vi "Set Setpoint.vi"(8 "error in":errorcluster, 10 "Setpoint":sgl, 11 "Alicat Controller in":refnum<class "Alicat Controller.lvclass">) -> (0 "error out":errorcluster, 3 "Alicat Controller out":refnum<class "Alicat Controller.lvclass">)   [LabVIEW 2015, in "Alicat.lvlib" / "Alicat Controller.lvclass"]
uses:
  Alicat Controller.lvclass
  Alicat Controller.lvclass/Alicat Controller.ctl
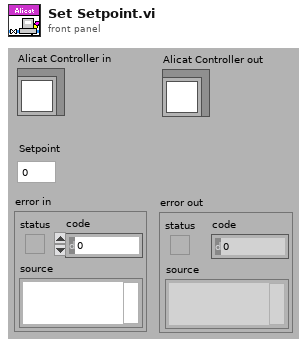
[diagram p1: front panel]
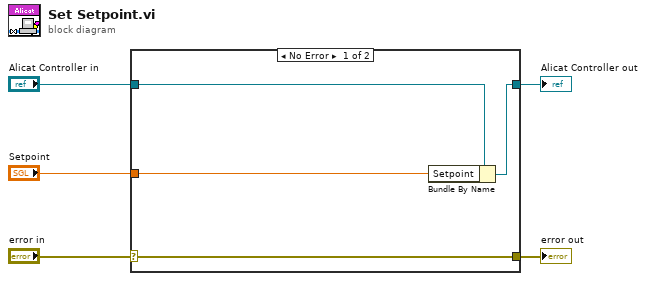
[diagram p0: block diagram]
diagram:
  n1 = case shown="No Error" "error in" {
    selector: "error in" -> [w9 w10]
    tunnel: [w9 w10] -> w4
    tunnel: [w7 w11] -> w2
    tunnel: "Alicat Controller in" -> [w8 w11]
    tunnel: "Setpoint" -> [w6 _]
    frame No Error {
      n2 = Bundle By Name(cluster=w8, "Setpoint"=w6) -> (w7:refnum<class "Alicat Controller.lvclass">)
    }
    frame Error {
    }
  }
  "error out" <- w4
  "Alicat Controller out" <- w2
